vi "Target Prosthesis Model.vi"(6 "Prosthesis Angle (degrees)":dbl, 9 "Lever Arm Polynomial":dbl[](array[numeric]) min=0.0 max=127.0 format="%#.2f", 10 "Spring Polynomial":dbl[](array[numeric]) min=0.0 max=127.0 format="%#.2f", 11 "Joint Torque Setpoint (Nm)":dbl) -> (0 "Force Setpoint (N)":dbl, 2 "Lever Arm (m)":dbl, 3 "Passive Torque (Nm)":dbl)   [LabVIEW 2018, in "COBRA Prosthesis Model Library.lvlib"]
uses:
  COBRA Prosthesis Model Library.lvlib
  <vilib>/Analysis/polynomials.llb/Scalar Polynomial Evaluation (DBL).vi
  <vilib>/Analysis/NI_AALPro.lvlib
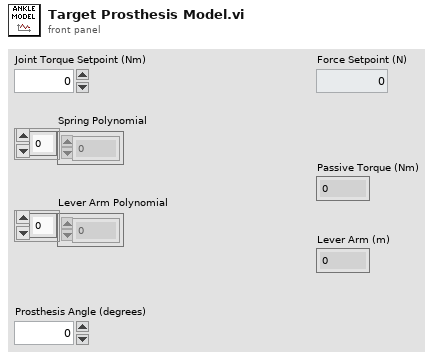
[diagram p1: front panel]
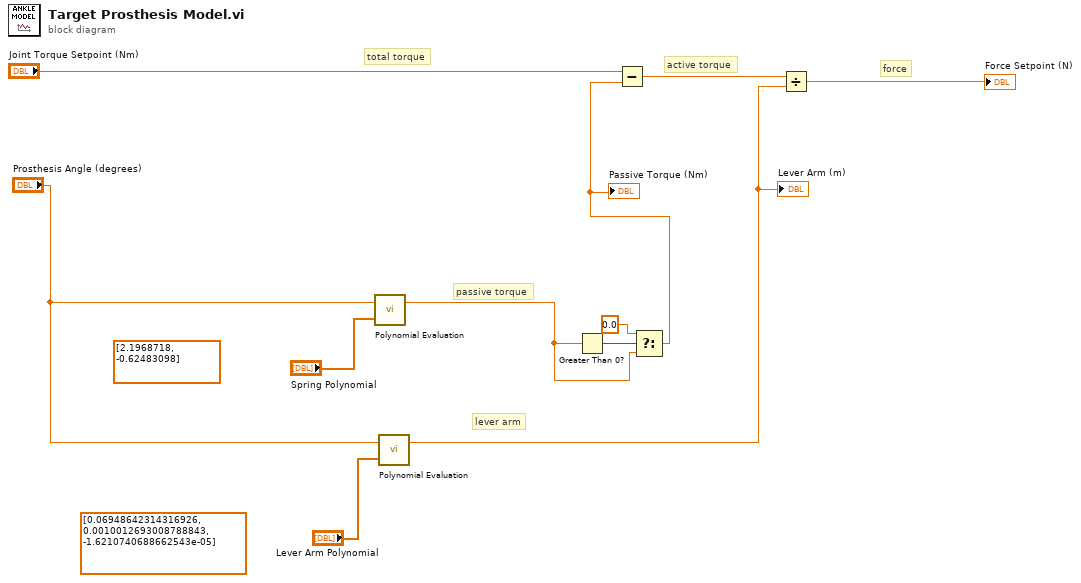
[diagram p0: block diagram]
diagram:
  (unwired) dbl[] [0.06948642314316926, 0.0010012693008788843, -1.6210740688662543e-05] ("P(x)")
  (unwired) dbl[] [2.1968718, -0.62483098] ("P(x)")
  # "lever arm"
  # "passive torque"
  # "total torque"
  # "force"
  # "active torque"
  n1 = call-poly <vilib>:"Polynomial Evaluation.vi"("P(x)"="Spring Polynomial", "a"="Prosthesis Angle (degrees)") -> ("P(a)"=w4:dbl)  [unwired: 1 out]
  n2 = call-poly <vilib>:"Polynomial Evaluation.vi"("P(x)"="Lever Arm Polynomial", "a"="Prosthesis Angle (degrees)") -> ("P(a)"=w7:dbl)  [unwired: 1 out]
  "Lever Arm (m)" <- w7
  n3 = Greater Than 0?(x=w4) -> (x > 0?=w6:bool)
  n4 = Select(t=0.0, s=w6, f=w4) -> (s? t:f=w3:dbl)
  "Passive Torque (Nm)" <- w3
  n5 = Subtract(x="Joint Torque Setpoint (Nm)", y=w3) -> (x-y=w10:dbl)
  n6 = Divide(x=w10, y=w7) -> (x/y=→"Force Setpoint (N)":dbl)
